vi "SR400 GetCountParams.vi"(8 "error in (no error)":errorcluster, 11 "VISA Port In":refnum<visa-resource-name>="SR400") -> (0 "error out":errorcluster, 1 "Dwell time":dbl=6.0 caption="\"Dwell Time\" (s)" min=0.002 max=6.0 step=0.001, 2 "Nb de période":i32=1 min=1 max=2000 step=1, 3 "VISA Port Out":refnum<visa-resource-name>="SR400", 4 "CounterPresT":dbl=0.001 caption="Counter T Preset (s)" min=1e-07 max=90000.0 step=1e-07 format="%#.7g", 5 "CounterPresB":dbl=0.001 caption="Counter B Preset (s)" min=1e-07 max=90000.0 step=1e-07 format="%#.7g", 7 "Mode":u16(ring) items=["A,B for T Preset", "A-B for T Preset", "A+B for T Preset", "A for B preset"])   [LabVIEW 2012]
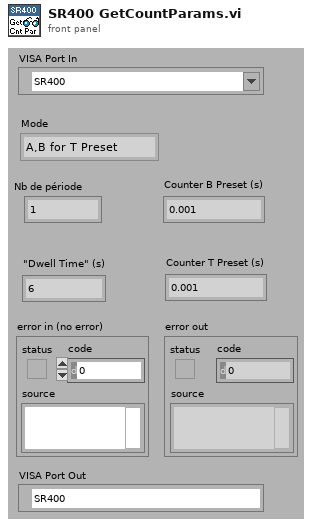
[diagram p1: front panel]
types:
  T1 = enum16{"Lit le Statut", "Demande Param", "Lit Param", "Oper. incomp."}
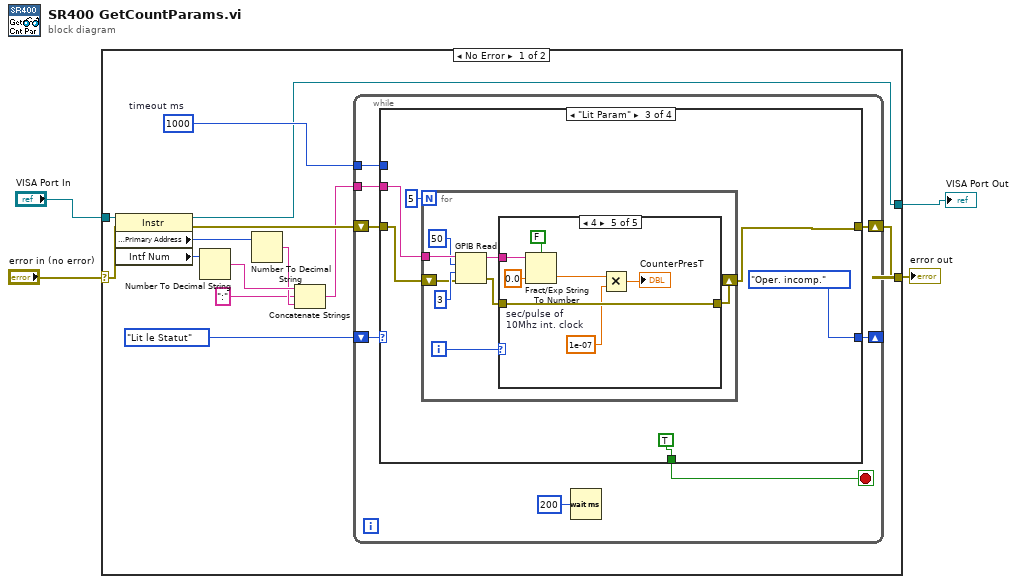
[diagram p0: block diagram]
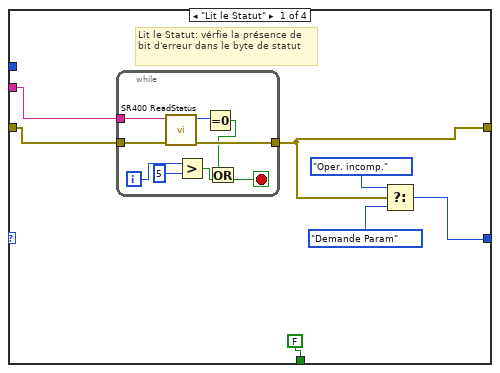
[diagram p2: hidden frame]
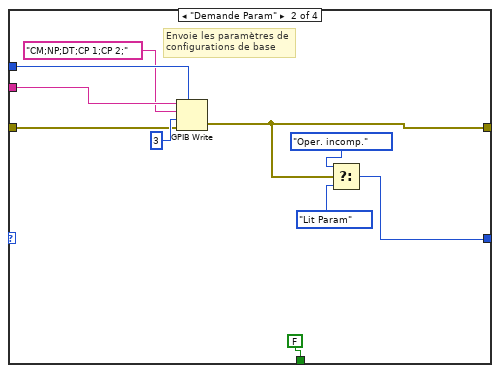
[diagram p3: hidden frame]
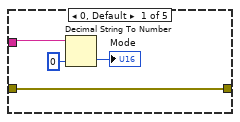
[diagram p4: hidden frame]
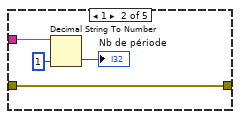
[diagram p5: hidden frame]
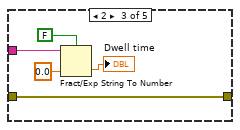
[diagram p6: hidden frame]
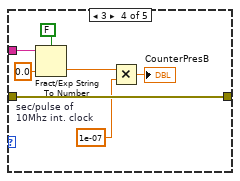
[diagram p7: hidden frame]
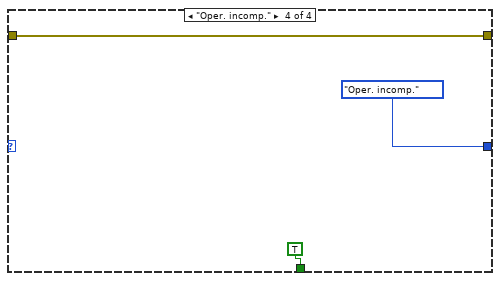
[diagram p8: hidden frame]
diagram:
  n1 = case shown="No Error" "error in (no error)" {
    selector: "error in (no error)" -> [w17 w97]
    tunnel: [w11 w97] -> w3
    tunnel: "VISA Port In" -> [w16 w96]
    tunnel: [w5 w96] -> w1
    frame No Error {
      w12 = 1000  # timeout ms
      n2 = property class="Instr"(reference=w16, error in=w17) -> (reference out=w5:refnum<visa-resource-name>, error out=w15:errorcluster, "GPIB Settings:Primary Address"=w13:u16, "Intf Num"=w10:u16)
      n3 = Number To Decimal String(number=w10) -> (decimal integer string=w9:string)  [unwired: 1 in]
      n4 = Number To Decimal String(number=w13) -> (decimal integer string=w8:string)  [unwired: 1 in]
      n5 = Concatenate Strings(w9, ":" ("string"), w8) -> (w6:string)
      n6 = while {
        shift-right: [w19] -> _
        shift-left: T1."Lit le Statut" -> [w25]
        tunnel: w6 -> [w23]
        shift-right: [w22] -> w11
        shift-left: w15 -> [w24]
        tunnel: w12 -> [w21]
        stop <- w20 stop-if-true
        n7 = case shown="\"Lit Param\"" w25 {
          tunnel: w24 -> [w31 w50 w54 w95]
          tunnel: w23 -> [w30 w49 w57 _]
          tunnel: [w26 w42 w52 w95] -> w22
          tunnel: w21 -> [_ w48 _ _]
          tunnel: [FALSE ("Configuration\neffectuée") FALSE ("Configuration\neffectuée") TRUE ("Configuration\neffectuée") TRUE ("Configuration\neffectuée")] -> w20
          tunnel: [w29 w46 T1."Oper. incomp." T1."Oper. incomp."] -> w19
          frame "Lit le Statut" {
            # "Lit le Statut: vérfie la présence de bit d'erreur dans le byte de statut"
            n8 = while {
              tunnel: w31 -> [w41]
              tunnel: w30 -> [w40]
              tunnel: [w39] -> w26
              i -> [w38]
              stop <- w35 stop-if-true
              n9 = call <userlib>:"SR400 ReadStatus.vi"("error in"=w41, "Address string"=w40) -> ("Error Out"=w39:errorcluster, "Status Code"=w34:u8)  [unwired: 6 in]
              n10 = Greater?(x=w38, y=5) -> (0:w36:bool)
              n11 = Equal To 0?(x=w34) -> (x = 0?=w33:bool)
              n12 = Or(x=w33, y=w36) -> (x .or. y?=w35:bool)
            }
            n13 = Select(t=T1."Oper. incomp.", s=w26, f=T1."Demande Param") -> (s? t:f=w29:T1)
          }
          frame "Demande Param" {
            # "Envoie les paramètres de configurations de base"
            n14 = GPIB Write(0:w49, 1:"CM;NP;DT;CP 1;CP 2;", 2:i16 3 ("mode (0)"), 3:w50, 4:w48) -> (6:w42:errorcluster)  [unwired: 1 out]
            n15 = Select(t=T1."Oper. incomp.", s=w42, f=T1."Lit Param") -> (s? t:f=w46:T1)
          }
          frame "Lit Param" {
            n16 = for {
              N: 5 -> [_]
              tunnel: w57 -> [w65]
              shift-right: [w58] -> w52
              shift-left: w54 -> [w62]
              i -> [w61]
              n17 = GPIB Read(0:w65, 1:50 ("byte count"), 2:i16 3 ("mode (0)"), 3:w62) -> (5:w60:string, 7:w59:errorcluster)  [unwired: 1 in, 1 out]
              n18 = case shown="4" w61 {
                tunnel: w60 -> [w69 w72 w76 w84 w91]
                tunnel: w59 -> [w66 w71 w75 w83 w90]
                tunnel: [w66 w71 w75 w83 w90] -> w58
                frame 0, Default {
                  n19 = Decimal String To Number(string=w69, default (0L)=u16 0 ("default (0 I32)")) -> (number=→"Mode":u16)  [unwired: 1 in, 1 out]
                }
                frame 1 {
                  n20 = Decimal String To Number(string=w72, default (0L)=1 ("default (0 I32)")) -> (number=→"Nb de période":i32)  [unwired: 1 in, 1 out]
                }
                frame 2 {
                  n21 = Fract/Exp String To Number(use system decimal point (T)=FALSE, string=w76, default (0 dbl)=0.0 ("default (0 I32)")) -> (number=→"Dwell time":dbl)  [unwired: 1 in, 1 out]
                }
                frame 3 {
                  w81 = 1e-07  # sec/pulse of 10Mhz int. clock
                  n22 = Fract/Exp String To Number(use system decimal point (T)=FALSE, string=w84, default (0 dbl)=0.0 ("default (0 I32)")) -> (number=w82:dbl)  [unwired: 1 in, 1 out]
                  n23 = Multiply(x=w82, y=w81) -> (x*y=→"CounterPresB":dbl)
                }
                frame 4 {
                  w88 = 1e-07  # sec/pulse of 10Mhz int. clock
                  n24 = Fract/Exp String To Number(use system decimal point (T)=FALSE, string=w91, default (0 dbl)=0.0 ("default (0 I32)")) -> (number=w89:dbl)  [unwired: 1 in, 1 out]
                  n25 = Multiply(x=w89, y=w88) -> (x*y=→"CounterPresT":dbl)
                }
              }
            }
          }
          frame "Oper. incomp." {
          }
        }
        n26 = Wait (ms)(milliseconds to wait=u32 200) -> ()  [unwired: 1 out]
      }
    }
    frame Error {
    }
  }
  "error out" <- w3
  "VISA Port Out" <- w1
